vi "ABR Main Panel.vi"(11 "State (in)":T16) -> (3 "State":T16)   [LabVIEW 2020]
uses:
  epl-vi-lib/Utility VIs/Buttons/KCheckmarkBoolean 2.ctl
  CFTS Main Panel SubVIs/CFTS-Experiment State.ctl
  TypeDefs/ABR-Analysis State.ctl
  Threshold Estimation VIs/ABR3-Threshold Estimation Result.ctl
  <vilib>/printing/EasyPrintingControls.llb/layout_options.ctl
  <vilib>/printing/EasyPrintingControls.llb/orientation.ctl
  <vilib>/printing/EasyPrintingControls.llb/panel_scaling_for_page.ctl
  <vilib>/printing/EasyPrintingControls.llb/margins.ctl
  <vilib>/printing/EasyPrintingControls.llb/margin_values.ctl
  <vilib>/printing/EasyPrintingControls.llb/measurement_system.ctl
  <vilib>/printing/EasyPrintingControls.llb/printer_options.ctl
  <vilib>/printing/EasyPrintingControls.llb/printing_method.ctl
  <vilib>/printing/EasyPrintingControls.llb/color_or_monochrome.ctl
  <vilib>/printing/EasyPrintingControls.llb/page_header_options.ctl
  <vilib>/printing/EasyPrintingControls.llb/page_headers.ctl
  <vilib>/printing/EasyPrintingControls.llb/page_header_content_options.ctl
  TypeDefs/ABR-Parameters.ctl
  TypeDefs/ABR-Stimulus.ctl
  TypeDefs/ABR-Response.ctl
  TypeDefs/ABR-Hidden Params.ctl
  Threshold Estimation VIs/ABR3-Threshold Estimation Parameters.ctl
  <vilib>/printing/EasyPrintingControls.llb/contents.ctl
  <vilib>/printing/EasyPrinting.llb/Easy Print VI Panel or Documentation (refnum).vi
  <vilib>/Utility/NIReport.llb/NI_ReportGenerationCore.lvlib
panel:
  out "Thr":string caption="Threshold (dB SPL)"
  in  "layout options":T1={"orientation (unchanged)"=0, "panel scaling for page (unchanged)"=0, "margins"={"override VI margins (false)"=FALSE, "margins (1.00)"={"top"=1.0, "left"=1.0, "right"=1.0, "bottom"=1.0}, "measurement system (default)"=0}, "printer options"={"destination printer name (current)"="", "printing method (unchanged)"=0, "color or monochrome (unchanged)"=0}, "page header options"={"page headers (unchanged)"=0, "page header content options"={"Include VI Name"=TRUE, "Include VI Path"=TRUE, "Include Last Modification Date"=TRUE, "Include Date Printed"=TRUE, "Include Page Number"=TRUE, "Include VI Icon"=TRUE}}} {"page header options"."page headers (unchanged)" items=["Unchanged", "Include page headers", "Do not include page headers"]; "printer options"."color or monochrome (unchanged)" items=["Unchanged", "Color/grayscale", "Monochrome"]; "printer options"."printing method (unchanged)" items=["Unchanged", "Standard", "PostScript", "Bitmap"]; "panel scaling for page (unchanged)" items=["Unchanged", "No Scaling", "Scale front panel to fit"]; "orientation (unchanged)" items=["Unchanged", "portrait", "landscape"]; "margins"."measurement system (default)" items=["Default", "US", "Metric"]; "margins"."margins (1.00)"."right" format="%.2f"; "margins"."margins (1.00)"."bottom" format="%.2f"; "margins"."margins (1.00)"."top" format="%.2f"; "margins"."margins (1.00)"."left" format="%.2f"}
  out "CM":cluster{dbl[], dbl[]}[](graph) caption="\"CM\""
  out "Neural":cluster{dbl[], dbl[]}[](graph)
  in  "NOTES":string
  out "Analysis":T13
  out "finished":errorcluster
  in  "Response":T15={"Gain"=10000, "Averages"=512, "Window (ms)"=8.5, "Thr Fast Steps"=1.5} {"Thr Fast Steps" format="%.2f"; "Window (ms)" format="%.2f"}
  in  "CAP or ABR":enum16{"CAP", "ABR"}(ring)=enum."ABR" caption="Measure what"
  out "MAX SPL":dbl=113.05999755859375 format="%.2f"
  out "SPL":dbl=35.0
  out "User":string
  out "Run #":u16=14
  out "ID #":u16=1
  out "Running":bool
  out "Abort":bool
  in  "Stimulus":T17={"Ear"=enum."Left", "Start (dB)"=20, "Waveform"=enum."TONE PIP", "Stop (dB)"=80, "Frequency (kHz)"=16.0, "Step (dB)"=5, "Rep rate (/sec)"=30.0, "Alternate Polarity"=FALSE} {"Rep rate (/sec)" format="%#_8g"; "Frequency (kHz)" format="%.2f"; "Start (dB)" step=5}
  out "Datafile":path
  in  "Normalize traces":T18=TRUE caption="Normalize individual traces"
  out "CLICK I-O":cluster{dbl[], dbl[]}[](graph)
  in  "START":bool
  in  "RETURN":bool
  in  "STOP":bool
  out "TONE I-O":cluster{dbl[], dbl[]}[](graph)
  # "Response"
  # "Running Average"
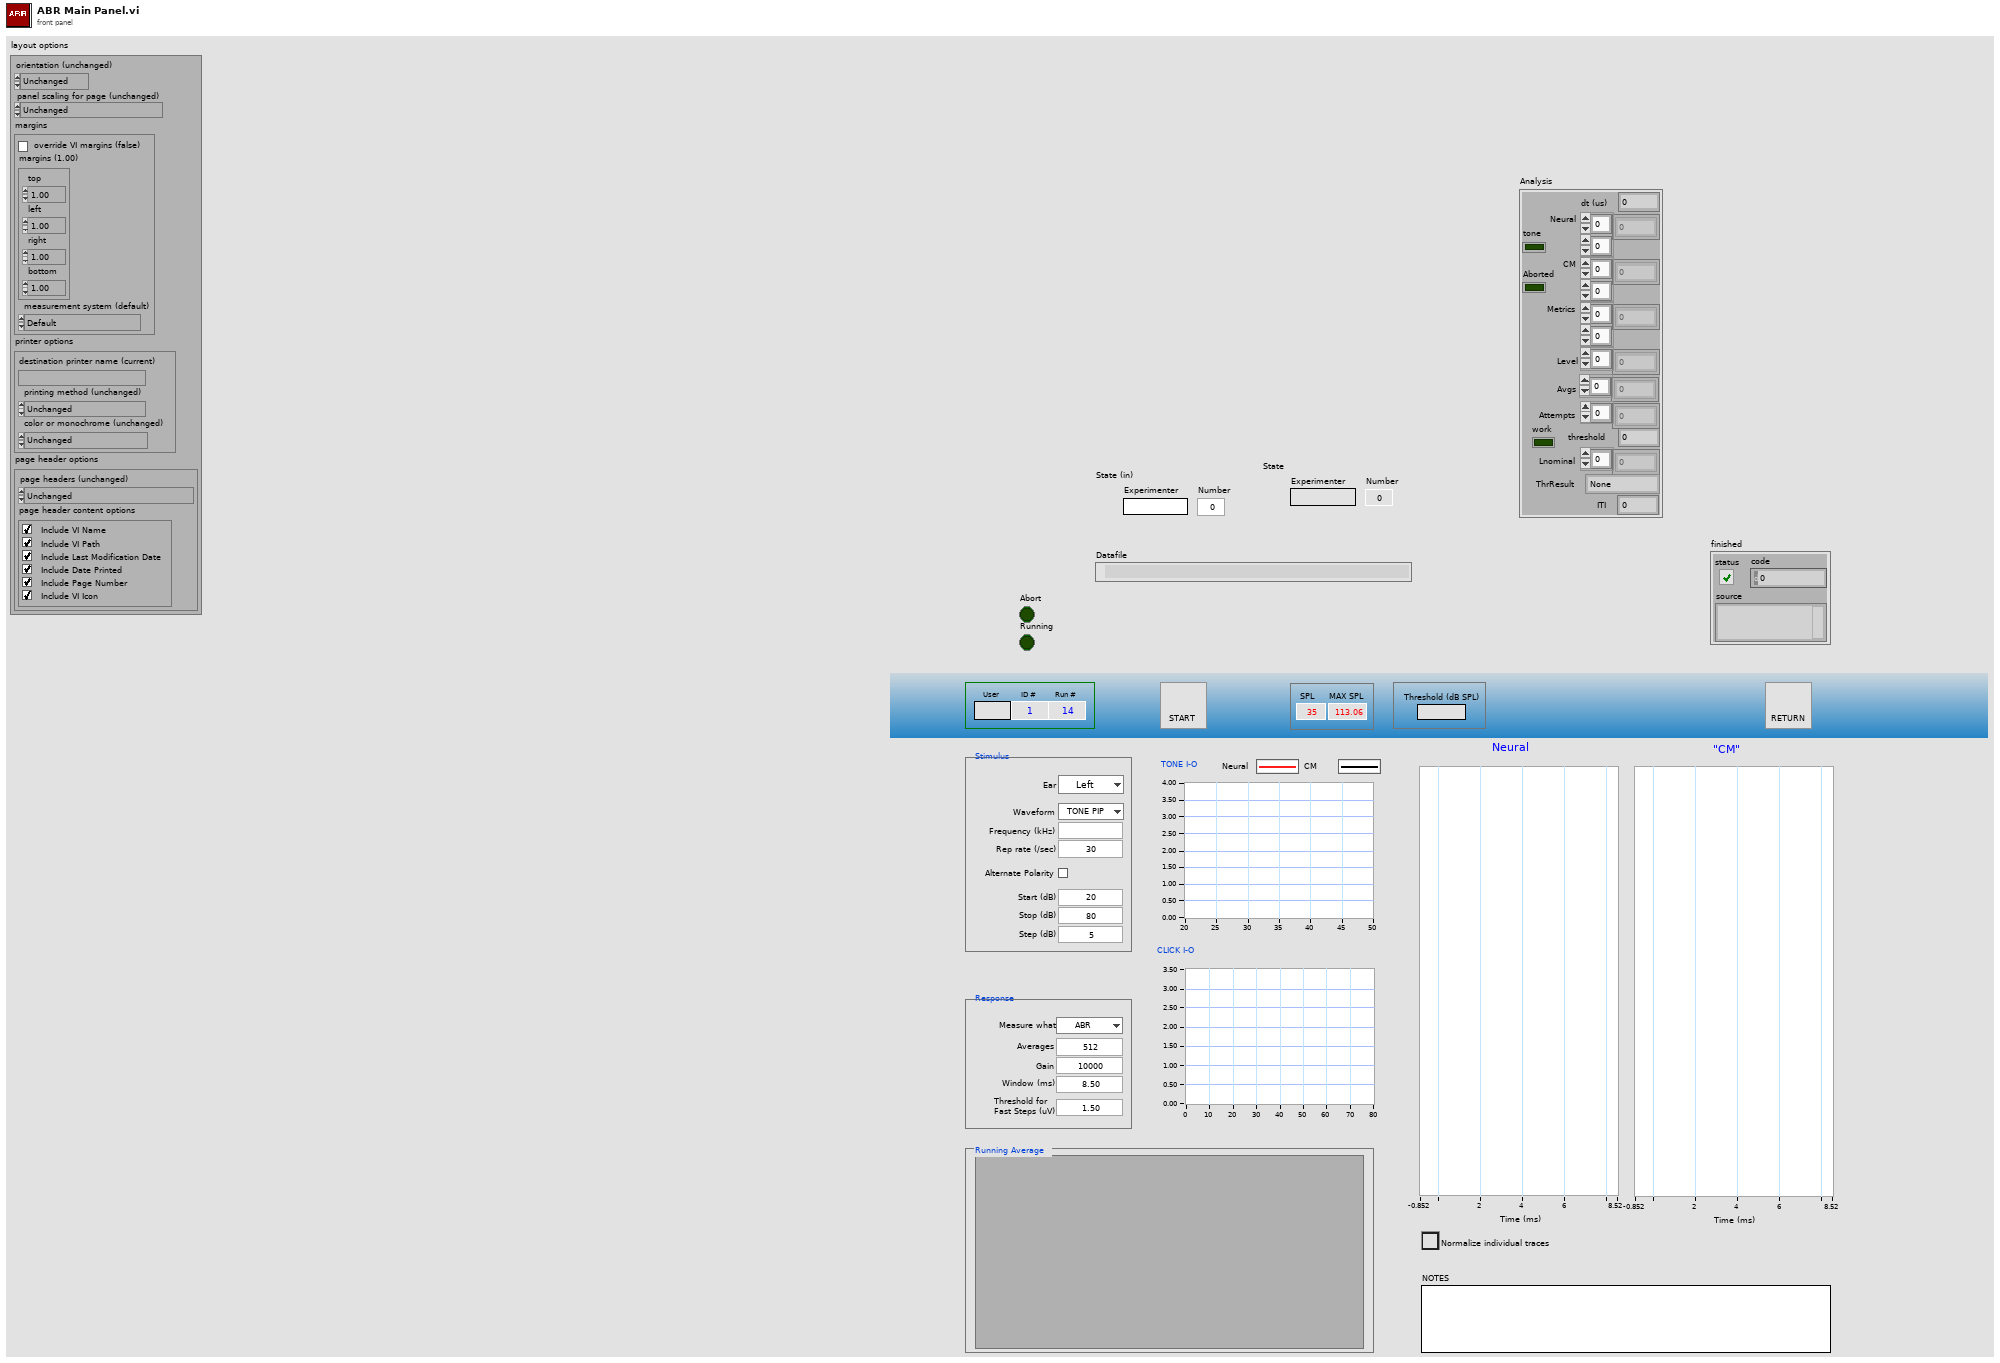
[diagram p1: front panel]
types:
  T1 = typedef "NI_ReportGenerationCore.lvlib/layout_options.ctl" = cluster{"orientation (unchanged)":T2, "panel scaling for page (unchanged)":T3, "margins":T4, "printer options":T7, "page header options":T10}
  T2 = typedef "NI_ReportGenerationCore.lvlib/orientation.ctl" = u16
  T3 = typedef "NI_ReportGenerationCore.lvlib/panel_scaling_for_page.ctl" = u16
  T4 = typedef "NI_ReportGenerationCore.lvlib/margins.ctl" = cluster{"override VI margins (false)":bool, "margins (1.00)":T5, "measurement system (default)":T6}
  T5 = typedef "NI_ReportGenerationCore.lvlib/margin_values.ctl" = cluster{"top":dbl, "left":dbl, "right":dbl, "bottom":dbl}
  T6 = typedef "NI_ReportGenerationCore.lvlib/measurement_system.ctl" = u16
  T7 = typedef "NI_ReportGenerationCore.lvlib/printer_options.ctl" = cluster{"destination printer name (current)":string, "printing method (unchanged)":T8, "color or monochrome (unchanged)":T9}
  T8 = typedef "NI_ReportGenerationCore.lvlib/printing_method.ctl" = u16
  T9 = typedef "NI_ReportGenerationCore.lvlib/color_or_monochrome.ctl" = u16
  T10 = typedef "NI_ReportGenerationCore.lvlib/page_header_options.ctl" = cluster{"page headers (unchanged)":T11, "page header content options":T12}
  T11 = typedef "NI_ReportGenerationCore.lvlib/page_headers.ctl" = u16
  T12 = typedef "NI_ReportGenerationCore.lvlib/page_header_content_options.ctl" = cluster{"Include VI Name":bool, "Include VI Path":bool, "Include Last Modification Date":bool, "Include Date Printed":bool, "Include Page Number":bool, "Include VI Icon":bool}
  T13 = typedef "ABR-Analysis State.ctl" = cluster{"dt (us)":dbl, "Neural":dbl[][], "CM":dbl[][], "Metrics":dbl[][], "Level":dbl[], "Avgs":i32[], "Attempts":i32[], "Aborted":bool, "threshold":dbl, "Lnominal":dbl[], "tone":bool, "work":bool, "ThrResult":T14, "ITI":dbl}
  T14 = typedef "ABR3-Threshold Estimation Result.ctl" = enum16{"None", "Power", "Sigmoid", "Power (noisy)", "Suprathreshold", "Invalid"}
  T15 = cluster{"Gain":i32, "Averages":i32, "Window (ms)":sgl, "Thr Fast Steps":sgl}
  T16 = typedef "CFTS-Experiment State.ctl" = cluster{"Experimenter":string, "Number":u32, "Right":string, "Left":string, "Data Folder":path, "State File":path, "Version Info":string, "End Exposure Time":dbl, "Exposure Duration":string, "Run #":cluster{"CAP":i16, "ABR":i16, "DP":i16, "VsEP":i16, "MeasSeq":i16, "SubSeq":i16, "SFOAE":i16}}
  T17 = cluster{"Ear":enum16{"Right", "Left"}, "Start (dB)":i32, "Waveform":enum16{"TONE PIP", "CLICK"}, "Stop (dB)":i32, "Frequency (kHz)":ext, "Step (dB)":i32, "Rep rate (/sec)":dbl, "Alternate Polarity":bool}
  T18 = typedef "KCheckmarkBoolean 2.ctl" = bool
  T19 = typedef "ABR3-Threshold Estimation Parameters.ctl" = cluster{"Tmin (ms)":dbl, "Tmax (ms)":dbl, "CC criterion":dbl, "adjR2 criterion":dbl}
  T20 = typedef "ABR-Parameters.ctl" = cluster{"CAP or ABR":enum16{"CAP", "ABR"}, "Stimulus":T21, "Response":T22, "Hidden":T23, "Version":i32}
  T21 = typedef "ABR-Stimulus.ctl" = cluster{"Ear":enum16{"Right", "Left", "Bone"}, "Start (dB)":i32, "Waveform":enum16{"TONE PIP", "CLICK"}, "Stop (dB)":i32, "Frequency (kHz)":ext, "Step (dB)":i32, "Rep rate (/sec)":dbl, "Alternate Polarity":bool}
  T22 = typedef "ABR-Response.ctl" = cluster{"Gain":i32, "Averages":i32, "Window (ms)":sgl, "Thr Fast Steps":sgl}
  T23 = typedef "ABR-Hidden Params.ctl" = cluster{"AI Samp Rate Hz":dbl, "AO Samp Rate Hz":dbl, "Duration (ms)":dbl, "Ramp (ms)":dbl, "Click width (us)":dbl, "ITI":enum16{"Rate", "Interval"}, "Save raw":bool}
  T24 = cluster{"Params":T20, "Threshold Estimation":T19}
  T25 = cluster{"TONE I-O":refnum<vi>, "Neural":refnum<vi>, "CM":refnum<vi>, "CLICK I-O":refnum<vi>}
  T26 = typedef "NI_ReportGenerationCore.lvlib/contents.ctl" = u16
  T27 = typedef "ABR3-Threshold Estimation Work.ctl" = cluster{"Threshold":dbl, "Criterion":dbl, "graphs":cluster{"X":dbl[], "Y":dbl[]}[], "Power2":string, "Sigmoid":string, "Result":T14}
  T28 = cluster{"Params":T20, "Threshold Estimation Out":T19}
  T29 = typedef "ABR-Runtime Data.ctl" = cluster{"AO Channels":i32[], "Ceiling":dbl, "Threshold":dbl, "Crossed?":bool, "Step":dbl, "Stop":i32, "Avgs":i32, "Level":dbl, "AI Npts":i32, "Doubled?":bool, "AO Npts":i32, "AltPol":bool, "dt":dbl, "gain":dbl, "reps/buffer":i32, "NWinPts":i32, "Save raw":bool}
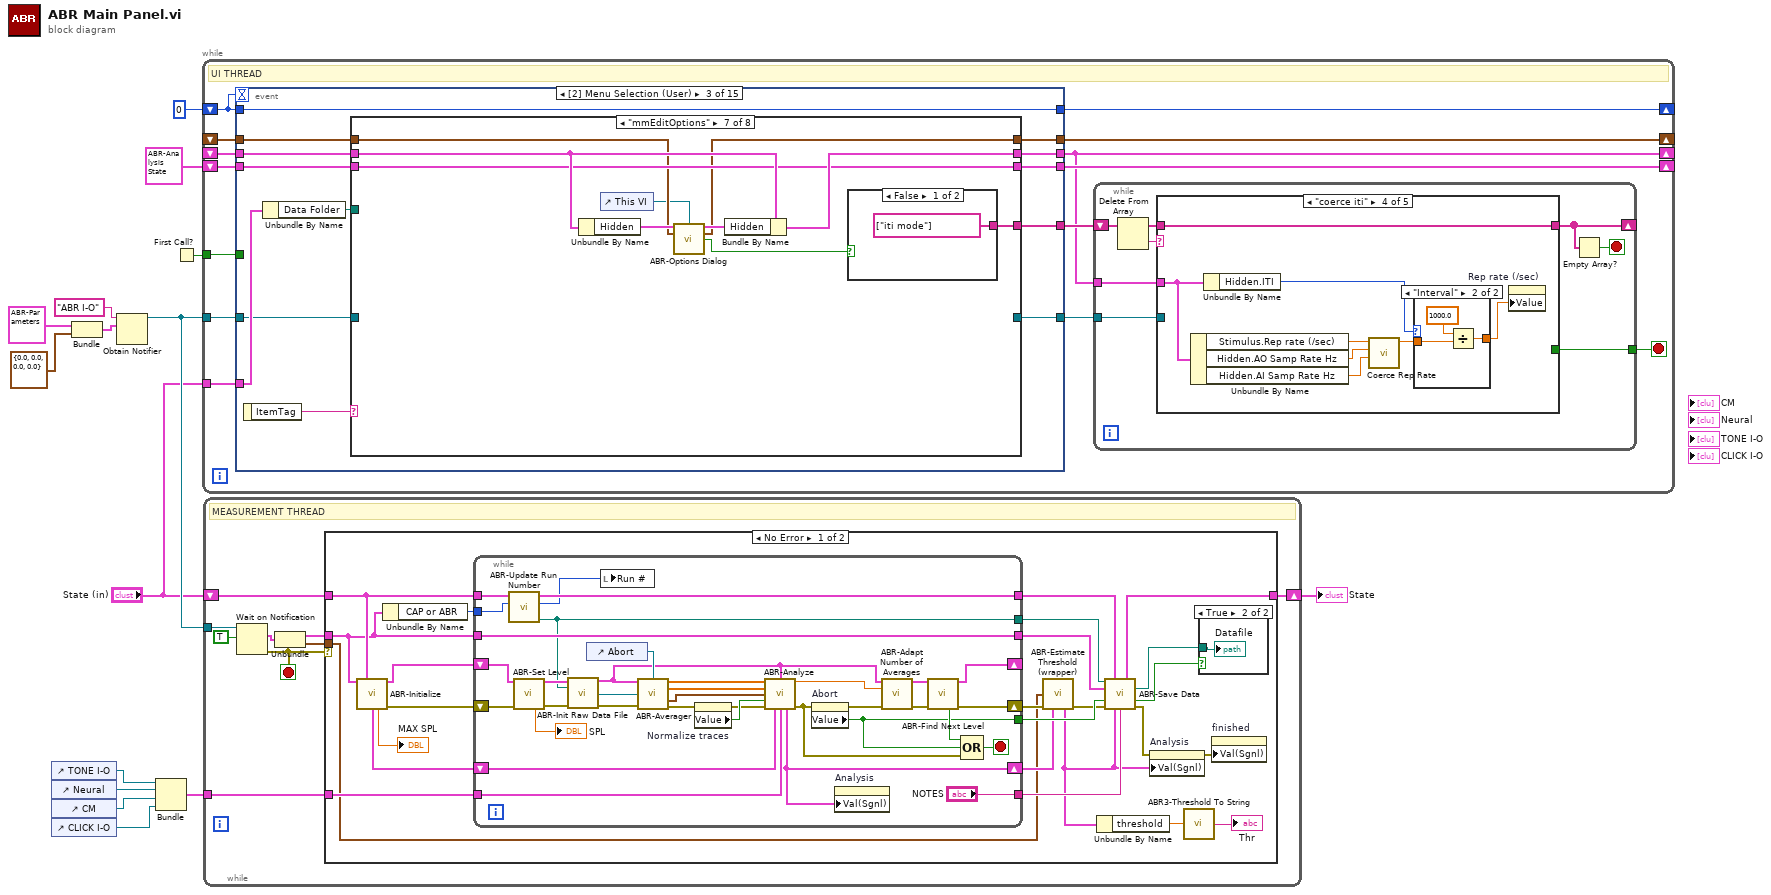
[diagram p0: block diagram]
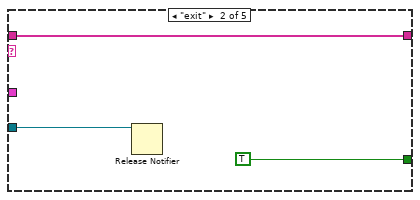
[diagram p5: hidden frame]
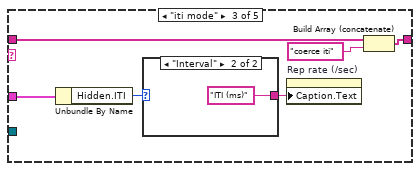
[diagram p6: hidden frame]
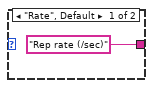
[diagram p7: hidden frame]
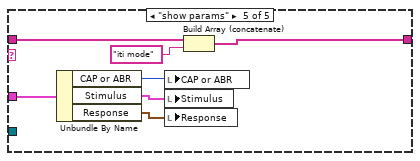
[diagram p9: hidden frame]
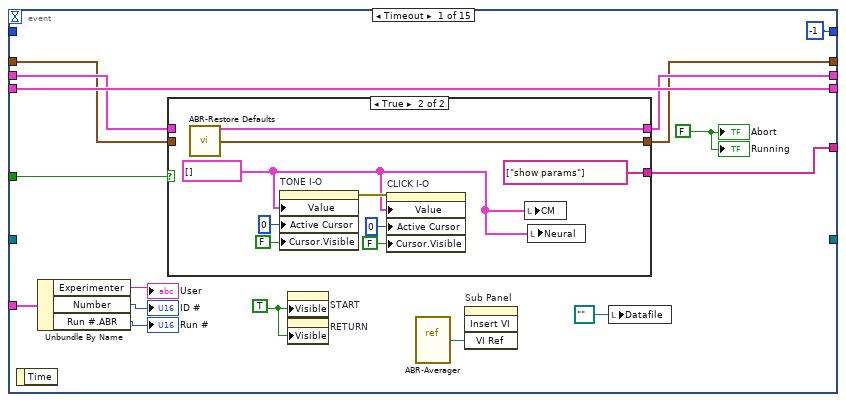
[diagram p10: hidden frame]
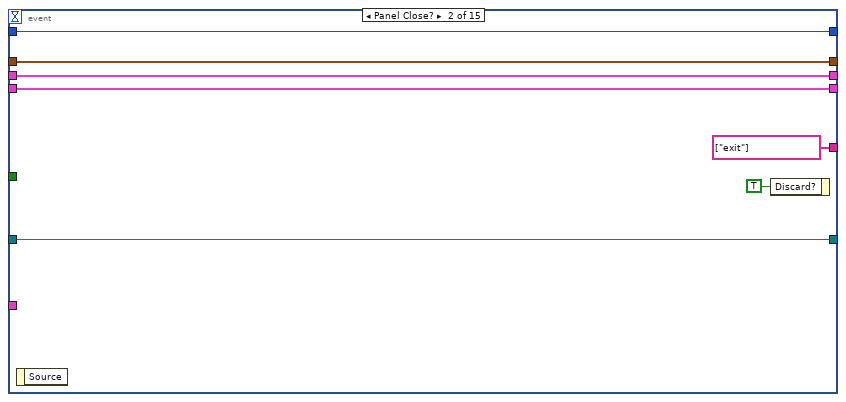
[diagram p12: hidden frame]
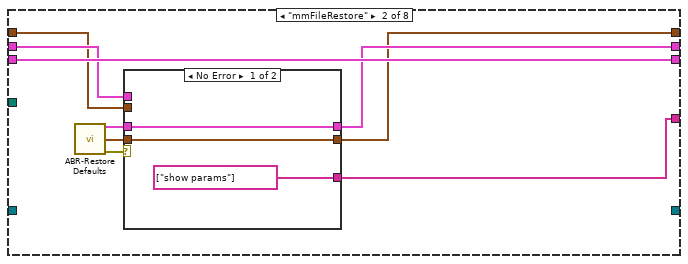
[diagram p14: hidden frame]
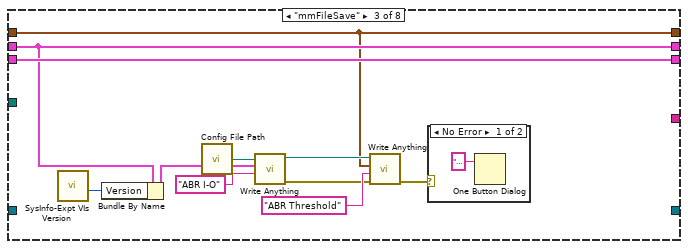
[diagram p16: hidden frame]
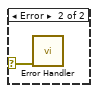
[diagram p17: hidden frame]
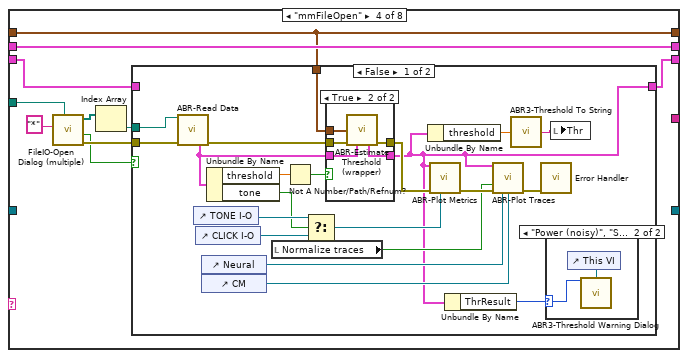
[diagram p18: hidden frame]
diagram:
  n1 = control-ref of="TONE I-O"() -> (w6:refnum<vi>)
  n2 = control-ref of="Neural"() -> (w8:refnum<vi>)
  n3 = control-ref of="CM"() -> (w7:refnum<vi>)
  n4 = control-ref of="CLICK I-O"() -> (w5:refnum<vi>)
  n5 = Bundle("Params"=T20 {"CAP or ABR"=enum."ABR", "Stimulus"={"Ear"=enum."Left", "Start (dB)"=0, "Waveform"=enum."TONE PIP", "Stop (dB)"=30, "Frequency (kHz)"=16.0, "Step (dB)"=5, "Rep rate (/sec)"=30.0, "Alternate Polarity"=FALSE}, "Response"={"Gain"=10000, "Averages"=512, "Window (ms)"=8.5, "Thr Fast Steps"=8.5}, "Hidden"={"AI Samp Rate Hz"=25000.0, "AO Samp Rate Hz"=100000.0, "Duration (ms)"=5.0, "Ramp (ms)"=0.5, "Click width (us)"=0.0, "ITI"=enum."Rate", "Save raw"=FALSE}, "Version"=0}, "Threshold Estimation"=T19 {"Tmin (ms)"=0.0, "Tmax (ms)"=0.0, "CC criterion"=0.0, "adjR2 criterion"=0.0}) -> (w1:T24)  [unwired: 1 in]
  n6 = Obtain Notifier(name (unnamed)="ABR I-O", notification data type=w1) -> (notifier out=w15:refnum<notifier>)  [unwired: 2 in, 2 out]
  n7 = Bundle("TONE I-O"=w6, "Neural"=w8, "CM"=w7, "CLICK I-O"=w5) -> (w9:T25)  [unwired: 1 in]
  n8 = First Call?() -> (First Call?: T/F=w13:bool)
  n9 = while {
    tunnel: w15 -> [w29]
    shift-right: [w26] -> _
    shift-left: 0 -> [w27]
    tunnel: w13 -> [w28]
    shift-right: [w17] -> _
    shift-left: _ -> [w25]
    tunnel: "State (in)" -> [w24]
    shift-right: [w22] -> _
    shift-left: T13 {"dt (us)"=0.0, "Neural"=[], "CM"=[], "Metrics"=[], "Level"=[], "Avgs"=[], "Attempts"=[], "Aborted"=FALSE, "threshold"=0.0, "Lnominal"=[], "tone"=FALSE, "work"=FALSE, "ThrResult"=enum."None", "ITI"=0.0} ("Analysis") -> [w23]
    shift-right: [w16] -> _
    shift-left: _ -> [w21]
    stop <- w18 stop-if-true
    # "UI THREAD"
    n10 = event shown="[2] Menu Selection (User)" {
      selector: _ -> [_ _ _ _ _ _ _ _ _ _ _ _ _ _ _]
      dyn-events: _ -> [_ _ _ _ _ _ _ _ _ _ _ _ _ _ _]
      timeout: w27 -> [_ _ _ _ _ _ _ _ _ _ _ _ _ _ _]
      tunnel: w29 -> [_ w96 w103 _ _ w230 w239 _ _ _ _ _ _ _ _]
      tunnel: [_ w96 w104 _ _ w230 _ _ _ _ _ _ _ _ _] -> w19
      tunnel: [-1 w102 w115 w218 w224 w229 w236 w243 w261 w267 w277 w299 w311 w317 w321] -> w26
      tunnel: w28 -> [w74 _ _ _ _ _ _ _ _ _ _ _ _ _ _]
      tunnel: w27 -> [_ w102 w115 w218 w224 w229 w236 w243 w261 w267 w277 w299 w311 w317 w321]
      tunnel: w25 -> [w73 w101 w111 w217 w223 w228 w232 w242 w258 w266 w276 w295 w310 w316 w320]
      tunnel: [w72 w101 w110 w217 w223 w228 w232 w242 w258 w266 w276 w298 w309 w315 w320] -> w17
      tunnel: w24 -> [w76 _ w113 _ _ _ _ _ _ _ _ _ _ _ _]
      tunnel: w23 -> [w75 w100 w109 w216 w222 w227 w235 w241 w247 w265 w275 w297 w307 w313 _]
      tunnel: [w75 w100 w108 w216 w221 w227 w235 w241 w247 w265 w275 w297 w307 w313 w319] -> w22
      tunnel: [w71 w98 w106 w213 w219 w226 w231 w240 w248 w264 w274 w296 w306 w312 w318] -> w16
      tunnel: w21 -> [w70 w98 w107 w213 w219 w226 w231 w240 w248 w264 w274 w296 w306 w312 w318]
      tunnel: [w69 string[] ["exit"] w105 _ _ string[] ["exit"] _ _ _ _ _ string[] ["coerce iti"] _ _ _] -> w20
      event Timeout {
        w79 = FALSE ("quitting")
        w80 = TRUE
        n11 = event-data() -> ()  [unwired: 1 in, 1 out]
        n12 = Unbundle By Name(w76) -> ("Experimenter"=→"User":string, "Number"=→"ID #":u32, "Run #.ABR"=→"Run #":i16)
        n13 = case shown="True" w74 {
          tunnel: w73 -> [w86 _]
          tunnel: [w86 w95] -> w72
          tunnel: [w85 w88] -> w71
          tunnel: w70 -> [w85 _]
          tunnel: [_ string[] ["show params"]] -> w69
          frame False {
          }
          frame True {
            w89 = cluster{dbl[], dbl[]}[] [] ("TONE I-O")
            n14 = call "ABR-Restore Defaults.vi"() -> ("Params"=w95:T20, "Threshold Estimation"=w88:T19)  [unwired: 13 in, 1 out]
            n15 = property on="TONE I-O" class="XYGraph (strict)"("Value"=w89, "Active Cursor"=u32 0, "Cursor.Visible"=FALSE) -> (error out=w92:errorcluster)  [unwired: 2 in, 1 out]
            n16 = property on="CLICK I-O" class="XYGraph (strict)"(error in=w92, "Value"=w89, "Active Cursor"=u32 0, "Cursor.Visible"=FALSE) -> ()  [unwired: 1 in, 2 out]
            n17 = local write "CM"(w89) -> ()
            n18 = local write "Neural"(w89) -> ()
          }
        }
        n19 = property on="START" class="Bool"("Visible"=w80) -> ()  [unwired: 2 in, 2 out]
        n20 = property on="RETURN" class="Bool"("Visible"=w80) -> ()  [unwired: 2 in, 2 out]
        n21 = vi-ref "ABR-Averager.vi"() -> (w83:refnum<vi>)
        n22 = invoke on="Sub Panel" class="SubPanel" method="Insert VI"("VI Ref"=w83) -> ()  [unwired: 3 in, 4 out]
        n23 = local write "Datafile"(path "" ("Datafile path")) -> ()
        "Abort" <- w79
        "Running" <- w79
      }
      event Panel Close? {
        n24 = event-data() -> ()  [unwired: 1 in, 1 out]
        n25 = event-data("Discard?"=TRUE) -> ()  [unwired: 1 in, 1 out]
      }
      event Menu Selection (User) {
        n26 = event-data() -> ("ItemTag"=w114:string)  [unwired: 1 in]
        n27 = Unbundle By Name(w113) -> ("Data Folder"=w112:path)
        n28 = case shown="\"mmEditOptions\"" w114 {
          tunnel: w111 -> [w118 w124 w141 w149 w192 w197 w204 w212]
          tunnel: [w118 w123 w141 w149 w192 w197 w205 w212] -> w110
          tunnel: w112 -> [_ _ _ w150 _ _ _ _]
          tunnel: w109 -> [w117 w127 w143 w148 w188 w196 w203 w210]
          tunnel: [w117 w127 w143 w147 w188 w196 w203 w210] -> w108
          tunnel: w107 -> [w116 w121 w135 w146 w187 w195 w202 w209]
          tunnel: [w116 w120 w135 w146 w187 w195 w201 w209] -> w106
          tunnel: [_ w119 _ _ _ string[] ["exit"] w198 _] -> w105
          tunnel: [_ _ _ _ _ w193 _ _] -> w104
          tunnel: w103 -> [_ _ _ _ _ w193 _ _]
          frame "False", Default {
          }
          frame "mmFileRestore" {
            n29 = call "ABR-Restore Defaults.vi"() -> ("Params"=w125:T20, "Threshold Estimation"=w122:T19, "error out"=w126:errorcluster)  [unwired: 13 in]
            n30 = case shown="No Error" w126 {
              tunnel: w125 -> [w130 _]
              tunnel: w124 -> [_ w132]
              tunnel: [w130 w132] -> w123
              tunnel: w122 -> [w129 _]
              tunnel: w121 -> [_ w131]
              tunnel: [w129 w131] -> w120
              tunnel: [string[] ["show params"] _] -> w119
              frame No Error {
              }
              frame Error {
              }
            }
          }
          frame "mmFileSave" {
            n31 = call "SysInfo-Expt VIs Version.vi"() -> ("Expt VIs Version out"=w133:i32)  [unwired: 11 in]
            n32 = Bundle By Name(cluster=w141, "Version"=w133) -> (w134:T20)
            n33 = call "Config File Path.vi"() -> ("Default config file name"=w142:path)  [unwired: 1 in]
            n34 = call "Write Anything.vi"("Section Name (Name of \"Anything\")"="ABR I-O" ("Section Name (Name of \"Anything\")"), "Anything"=w134, "Path (dialog)"=w142) -> ("Error Out"=w137:errorcluster, "Path out"=w138:path)  [unwired: 7 in]
            n35 = call "Write Anything.vi"("Error In"=w137, "Section Name (Name of \"Anything\")"="ABR Threshold" ("Section Name (Name of \"Anything\")"), "Anything"=w135, "Path (dialog)"=w138) -> ("Error Out"=w136:errorcluster)  [unwired: 6 in, 1 out]
            n36 = case shown="No Error" w136 {
              selector: w136 -> [_ w145]
              frame No Error {
                n37 = One Button Dialog(message="Defaults saved.") -> ()  [unwired: 1 in, 1 out]
              }
              frame Error {
                n38 = call "Error Handler.vi"("error in (no error)"=w145) -> ()  [unwired: 13 in, 2 out]
              }
            }
          }
          frame "mmFileOpen" {
            n39 = call "FileIO-Open Dialog (multiple).vi"("Default Folder"=w150, "pattern (all files)"="*") -> ("error out"=w155:errorcluster, "cancelled"=w151:bool, "Paths"=w154:path[])  [unwired: 7 in]
            n40 = Index Array(array=w154) -> (element=w153:path)  [unwired: 1 in]
            n41 = case shown="False" w151 {
              tunnel: w155 -> [w176 _]
              tunnel: w153 -> [w175 _]
              tunnel: w148 -> [_ w186]
              tunnel: [w157 w186] -> w147
              tunnel: w146 -> [w158 _]
              frame False {
                n42 = call "ABR-Read Data.vi"("Path"=w175, "error in (no error)"=w176) -> ("Analysis"=w161:T13, "error out"=w163:errorcluster)  [unwired: 8 in, 4 out]
                n43 = control-ref of="TONE I-O"() -> (w168:refnum<vi>)
                n44 = control-ref of="CLICK I-O"() -> (w169:refnum<vi>)
                n45 = control-ref of="Neural"() -> (w172:refnum<vi>)
                n46 = control-ref of="CM"() -> (w171:refnum<vi>)
                n47 = Unbundle By Name(w161) -> ("threshold"=w165:dbl, "tone"=w166:bool)
                n48 = local read "Normalize traces"() -> (w173:T18)
                n49 = Not A Number/Path/Refnum?(number/path/refnum=w165) -> (NaN/Path/Refnum?=w164:bool)
                n50 = Select(t=w168, s=w166, f=w169) -> (s? t:f=w167:refnum<vi>)
                n51 = case shown="True" w164 {
                  tunnel: w163 -> [w180 w185]
                  tunnel: [w180 w184] -> w162
                  tunnel: w161 -> [w179 w183]
                  tunnel: [w179 w182] -> w157
                  tunnel: w158 -> [_ w181]
                  frame False {
                  }
                  frame True {
                    n52 = call "ABR-Estimate Threshold (wrapper).vi"("Threshold Estimation"=w181, "error in (no error)"=w185, "Analysis (in)"=w183) -> ("Analysis (out)"=w182:T13, "error out"=w184:errorcluster)  [unwired: 10 in, 1 out]
                  }
                }
                n53 = Unbundle By Name(w157) -> ("threshold"=w160:dbl)
                n54 = call "ABR-Plot Metrics.vi"("Analysis"=w157, "error in (no error)"=w162, "I-O"=w167) -> ("error out"=w174:errorcluster)  [unwired: 12 in]
                n55 = Unbundle By Name(w157) -> ("ThrResult"=w156:T14)
                n56 = call "ABR-Plot Traces.vi"("Analysis"=w157, "Normalize individual?"=w173, "error in (no error)"=w174, "Neural Ref"=w172, "CM Ref"=w171) -> ("error out"=w170:errorcluster)  [unwired: 10 in]
                n57 = call "ABR3-Threshold To String.vi"("Threshold"=w160) -> ("String"=w159:string)
                n58 = call "Error Handler.vi"("error in (no error)"=w170) -> ()  [unwired: 13 in, 2 out]
                n59 = case shown="\"Power (noisy)\", \"Suprathreshold\"" w156 {
                  selector: w156 -> [_ w178]
                  frame "None", Default {
                  }
                  frame "Power (noisy)", "Suprathreshold" {
                    n60 = control-ref of="This VI"() -> (w177:refnum<vi>)
                    n61 = call "ABR3-Threshold Warning Dialog.vi"("Result"=w178, "Parent VI"=w177) -> ()  [unwired: 14 in]
                  }
                }
                n62 = local write "Thr"(w159) -> ()
              }
              frame True {
              }
            }
          }
          frame "mmFilePrint" {
            w191 = T26 1 items=["Complete front panel", "Visible portion of front panel", "Icon, description, panel and diagram", "Documentation: Using the panel", "Documentation: Using as a subVI", "Documentation: Complete", "Documentation: Custom"] ("contents (complete front panel)")
            n63 = control-ref of="This VI"() -> (w189:refnum<vi>)
            n64 = call-poly <vilib>:"Easy Print VI Panel or Documentation.vi"("layout options"="layout options", "contents (complete front panel)"=w191, "VI reference"=w189) -> ()  [unwired: 7 in, 2 out]
          }
          frame "mmFileExit" {
          }
          frame "mmEditOptions" {
            n65 = Unbundle By Name(w204) -> ("Hidden"=w207:T23)
            n66 = control-ref of="This VI"() -> (w200:refnum<vi>)
            n67 = call "ABR-Options Dialog.vi"("Hidden"=w207, "Parent VI"=w200, "Threshold Estimation In"=w202) -> ("Cluster out"=w206:T23, "Threshold Estimation Out"=w201:T19, "Canceled?"=w199:bool)  [unwired: 10 in]
            n68 = Bundle By Name(cluster=w204, "Hidden"=w206) -> (w205:T20)
            n69 = case shown="False" w199 {
              tunnel: [string[] ["iti mode"] _] -> w198
              frame False {
              }
              frame True {
              }
            }
          }
          frame "mmHelpManual" {
            n70 = call "CFTS-Open Help Topic.vi"("Topic Keyword"="ABR/CAP") -> ()  [unwired: 14 in, 1 out]
          }
        }
      }
      event "CLICK I-O", "TONE I-O": Shortcut Menu Activation? {
        n71 = event-data() -> ()  [unwired: 1 in, 1 out]
        n72 = Unbundle By Name(w216) -> ("Neural"=w215:dbl[][])
        n73 = Empty Array?(array=w215) -> (empty?=w214:bool)
        n74 = event-data("Discard?"=w214) -> ()  [unwired: 1 in, 1 out]
      }
      event "CLICK I-O", "TONE I-O": Shortcut Menu Selection (User) {
        n75 = event-data() -> ()  [unwired: 1 in, 1 out]
        n76 = call "ABR-Estimate Threshold (wrapper).vi"("Analysis (in)"=w222) -> ("Work"=w220:T27, "Analysis (out)"=w221:T13)  [unwired: 12 in, 1 out]
        n77 = call "ABR3-Show Threshold Estimation Work.vi"("work"=w220) -> ()  [unwired: 15 in]
      }
      event "RETURN": Value Change {
        n78 = event-data() -> ()  [unwired: 1 in, 1 out]
      }
      event "START": Value Change {
        w237 = FALSE ("ABI Abort")
        n79 = event-data() -> ()  [unwired: 1 in, 1 out]
        n80 = Bundle("Params"=w232, "Threshold Estimation Out"=w231) -> (w233:T28)  [unwired: 1 in]
        n81 = Send Notification(notification=w233, notifier=w239) -> ()  [unwired: 1 in, 2 out]
        n82 = local write "NOTES"("" ("NOTES")) -> ()
        n83 = local write "Abort"(w237) -> ()
        n84 = property on="RETURN" class="Bool"("Visible"=w237) -> ()  [unwired: 2 in, 2 out]
        n85 = property on="START" class="Bool"("Visible"=w237) -> ()  [unwired: 2 in, 2 out]
        n86 = local write "Running"(TRUE ("Running")) -> ()
      }
      event "STOP": Value Change {
        n87 = event-data() -> ()  [unwired: 1 in, 1 out]
        n88 = local write "Abort"(TRUE ("Stopping")) -> ()
      }
      event "finished": Value Change {
        w259 = TRUE
        n89 = event-data() -> ("NewVal"=w257:errorcluster)  [unwired: 1 in]
        n90 = Unbundle By Name(w247) -> ("tone"=w256:bool)
        n91 = call "Error Handler.vi"("error in (no error)"=w257) -> ()  [unwired: 13 in, 2 out]
        n92 = control-ref of="TONE I-O"() -> (w254:refnum<vi>)
        n93 = control-ref of="CLICK I-O"() -> (w253:refnum<vi>)
        n94 = control-ref of="Neural"() -> (w251:refnum<vi>)
        n95 = control-ref of="CM"() -> (w252:refnum<vi>)
        n96 = local read "Normalize traces"() -> (w250:T18)
        n97 = Select(t=w254, s=w256, f=w253) -> (s? t:f=w255:refnum<vi>)
        n98 = call "ABR-Plot Metrics.vi"("Analysis"=w247, "I-O"=w255) -> ("error out"=w249:errorcluster)  [unwired: 13 in]
        n99 = Unbundle By Name(w247) -> ("ThrResult"=w246:T14)
        n100 = call "ABR-Plot Traces.vi"("Analysis"=w247, "Normalize individual?"=w250, "error in (no error)"=w249, "Neural Ref"=w251, "CM Ref"=w252) -> ("error out"=w245:errorcluster)  [unwired: 10 in]
        n101 = case shown="\"Power (noisy)\", \"Suprathreshold\"" w246 {
          selector: w246 -> [_ w263]
          tunnel: w245 -> [_ _]
          frame "None", Default {
          }
          frame "Power (noisy)", "Suprathreshold" {
            n102 = control-ref of="This VI"() -> (w262:refnum<vi>)
            n103 = call "ABR3-Threshold Warning Dialog.vi"("Result"=w263, "Parent VI"=w262) -> ()  [unwired: 14 in]
          }
        }
        n104 = call "Beeper.vi"() -> ()  [unwired: 5 in, 1 out]
        n105 = property on="RETURN" class="Bool"("Visible"=w259) -> ()  [unwired: 2 in, 2 out]
        n106 = property on="START" class="Bool"("Visible"=w259) -> ()  [unwired: 2 in, 2 out]
        n107 = local write "Running"(FALSE ("Running")) -> ()
      }
      event Value Change {
        n108 = event-data() -> ("NewVal"=w269:T18)  [unwired: 1 in]
        n109 = case shown="False" FALSE {
          tunnel: w269 -> [w273 _]
          tunnel: w265 -> [w272 _]
          frame False {
            n110 = control-ref of="Neural"() -> (w271:refnum<vi>)
            n111 = control-ref of="CM"() -> (w270:refnum<vi>)
            n112 = call "ABR-Plot Traces.vi"("Analysis"=w272, "Normalize individual?"=w273, "Neural Ref"=w271, "CM Ref"=w270) -> ()  [unwired: 11 in, 1 out]
          }
          frame True {
          }
        }
      }
      event "NOTES": Value Change {
        n113 = event-data() -> ("NewVal"=w279:string)  [unwired: 1 in]
        n114 = local read "Running"() -> (w285:bool)
        n115 = local read "Datafile"() -> (w280:path)
        n116 = Not(x=w285) -> (.not. x?=w283:bool)
        n117 = Empty String/Path?(string/path=w280) -> (empty?=w284:bool)
        n118 = Not(x=w284) -> (.not. x?=w282:bool)
        n119 = And(x=w282, y=w283) -> (x .and. y?=w281:bool)
        n120 = case shown="True" w281 {
          tunnel: w280 -> [_ w289]
          tunnel: w279 -> [_ w288]
          tunnel: "Add notes to data file?" ("message") -> [_ w287]
          frame False {
          }
          frame True {
            n121 = Two Button Dialog(message=w287) -> (T button?=w286:bool)  [unwired: 2 in]
            n122 = case shown="True" w286 {
              tunnel: w289 -> [_ w290]
              tunnel: w288 -> [_ _]
              frame False {
              }
              frame True {
                n123 = call "ABR-Insert Notes.vi"("path"=w290) -> ()  [unwired: 13 in, 2 out]
              }
            }
          }
        }
      }
      event "Stimulus": Value Change {
        n124 = event-data() -> ()  [unwired: 1 in, 1 out]
        n125 = Unbundle By Name(w295) -> ("Hidden.ITI"=w294:enum16{"Rate", "Interval"})
        n126 = case shown="\"Interval\"" w294 {
          tunnel: [w300 w301] -> w293
          tunnel: "Stimulus" -> [w300 w303]
          frame "Rate", Default {
          }
          frame "Interval" {
            n127 = Unbundle By Name(w303) -> ("Rep rate (/sec)"=w305:dbl)
            n128 = Divide(x=1000.0, y=w305) -> (x/y=w302:dbl)
            n129 = Bundle By Name(cluster=w303, "Rep rate (/sec)"=w302) -> (w301:T17)
          }
        }
        n130 = Bundle By Name(cluster=w295, "Stimulus"=w293) -> (w298:T20)
      }
      event "CAP or ABR": Value Change {
        n131 = event-data() -> ()  [unwired: 1 in, 1 out]
        n132 = Bundle By Name(cluster=w310, "CAP or ABR"="CAP or ABR") -> (w309:T20)
      }
      event "Response": Value Change {
        n133 = event-data() -> ()  [unwired: 1 in, 1 out]
        n134 = Bundle By Name(cluster=w316, "Response"="Response") -> (w315:T20)
      }
      event Value Change {
        n135 = event-data() -> ("NewVal"=w319:T13)  [unwired: 1 in]
      }
    }
    n136 = while {
      shift-right: [w34] -> _
      shift-left: w20 -> [w37]
      tunnel: w19 -> [w32]
      tunnel: [w31] -> w18
      tunnel: w17 -> [w30]
      stop <- w33 stop-if-true
      n137 = Delete From Array(array=w37) -> (deleted portion=w35:string, array with subset deleted=w36:string[])  [unwired: 2 in]
      n138 = case shown="\"coerce iti\"" w35 {
        tunnel: w36 -> [w38 w41 w47 w57 w68]
        tunnel: [w38 w41 w43 w57 w63] -> w34
        tunnel: w32 -> [_ w40 _ _ _]
        tunnel: [_ TRUE _ _ _] -> w31
        tunnel: w30 -> [_ _ w46 w55 w64]
        frame "", Default {
        }
        frame "exit" {
          n139 = Release Notifier(notifier=w40) -> ()  [unwired: 2 in, 3 out]
        }
        frame "iti mode" {
          n140 = Unbundle By Name(w46) -> ("Hidden.ITI"=w45:enum16{"Rate", "Interval"})
          n141 = case shown="\"Interval\"" w45 {
            tunnel: ["Rep rate (/sec)" ("Caption.Text") "ITI (ms)" ("Caption.Text")] -> w44
            frame "Rate", Default {
            }
            frame "Interval" {
            }
          }
          n142 = property on="Rep rate (/sec)" class="DigNum (strict)"("Caption.Text"=w44) -> ()  [unwired: 2 in, 2 out]
          n143 = Build Array (concatenate)(w47, "coerce iti") -> (w43:string[])
        }
        frame "coerce iti" {
          n144 = Unbundle By Name(w55) -> ("Stimulus.Rep rate (/sec)"=w54:dbl, "Hidden.AO Samp Rate Hz"=w53:dbl, "Hidden.AI Samp Rate Hz"=w52:dbl)
          n145 = Unbundle By Name(w55) -> ("Hidden.ITI"=w56:enum16{"Rate", "Interval"})
          n146 = call "Coerce Rep Rate.vi"("AI sampling rate (Hz)"=w52, "AO sampling rate (Hz)"=w53, "Rep rate (Hz)"=w54) -> ("Coerced rep rate (Hz)"=w51:dbl)  [unwired: 5 in, 3 out]
          n147 = case shown="\"Interval\"" w56 {
            tunnel: w51 -> [w58 w61]
            tunnel: [w58 w60] -> w50
            frame "Rate", Default {
            }
            frame "Interval" {
              n148 = Divide(x=1000.0, y=w61) -> (x/y=w60:dbl)
            }
          }
          n149 = property on="Rep rate (/sec)" class="DigNum (strict)"("Value"=w50) -> ()  [unwired: 2 in, 2 out]
        }
        frame "show params" {
          n150 = Unbundle By Name(w64) -> ("CAP or ABR"=w67:enum16{"CAP", "ABR"}, "Stimulus"=w66:T21, "Response"=w65:T22)
          n151 = local write "CAP or ABR"(w67) -> ()
          n152 = local write "Stimulus"(w66) -> ()
          n153 = local write "Response"(w65) -> ()
          n154 = Build Array (concatenate)(w68, "iti mode") -> (w63:string[])
        }
      }
      n155 = Empty Array?(array=w34) -> (empty?=w33:bool)
    }
  }
  n156 = while {
    tunnel: w15 -> [w329]
    shift-right: [w325] -> w10
    shift-left: "State (in)" -> [w326]
    tunnel: w9 -> [w324]
    stop <- w328 stop-if-true
    # "MEASUREMENT THREAD"
    n157 = Wait on Notification(notifier=w329, ignore previous (F)=TRUE) -> (notification=w327:T24, error out=w328:errorcluster)  [unwired: 2 in, 2 out]
    n158 = Unbundle(w327) -> ("Params"=w323:T20, "Threshold Estimation"=w322:T19)
    n159 = case shown="No Error" w328 {
      tunnel: w323 -> [w342 _]
      tunnel: w326 -> [w352 w392]
      tunnel: [w348 w392] -> w325
      tunnel: w324 -> [w350 _]
      tunnel: w322 -> [w332 _]
      frame No Error {
        n160 = call "ABR-Initialize.vi"("Params"=w342, "State"=w352) -> ("Runtime"=w354:T29, "Analysis"=w351:T13, "Ceiling"=→"MAX SPL":dbl, "error out"=w355:errorcluster)  [unwired: 10 in]
        n161 = Unbundle By Name(w342) -> ("CAP or ABR"=w341:enum16{"CAP", "ABR"})
        n162 = while {
          shift-right: [w389] -> w340
          shift-left: w355 -> [w387]
          shift-right: [w385] -> _
          shift-left: w354 -> [w384]
          tunnel: w352 -> [w382]
          tunnel: [w381] -> w349
          shift-right: [w365] -> w338
          shift-left: w351 -> [w375]
          tunnel: w350 -> [w374]
          tunnel: ["NOTES"] -> w347
          tunnel: [w367] -> w346
          tunnel: [w366] -> w343
          tunnel: w342 -> [w366]
          tunnel: w341 -> [w364]
          tunnel: [w357] -> w331
          stop <- w391 stop-if-true
          # "stepsize"
          # "max SPL"
          # "array of levels"
          # "current SPL"
          n163 = call "ABR-Update Run Number.vi"("CAP or ABR"=w364, "State (in)"=w382) -> ("raw data filestem"=w357:path, "run #"=w358:i16, "State (out)"=w381:T16)  [unwired: 7 in]
          n164 = call "ABR-Set Level.vi"("Runtime"=w384, "error in (no error)"=w387) -> ("Runtime out"=w363:T29, "Level"=→"SPL":dbl, "error out"=w361:errorcluster)  [unwired: 11 in]
          n165 = call "ABR-Init Raw Data File.vi"("Runtime in"=w363, "Path"=w357, "error in (no error)"=w361) -> ("Runtime out"=w362:T29, "refnum out"=w359:refnum<file>, "error out"=w360:errorcluster)  [unwired: 10 in]
          n166 = control-ref of="Abort"() -> (w390:refnum<vi>)
          n167 = local write "Run #"(w358) -> ()
          n168 = call "ABR-Averager.vi"("Runtime"=w362, "Abort"=w390, "raw data file"=w359, "error in (no error)"=w360) -> ("Neural (uV)"=w380:dbl[], "microphonic (uV)"=w379:dbl[], "Averaging data"=w378:cluster{i32, i32}, "error out"=w383:errorcluster)  [unwired: 8 in]
          n169 = property on="Normalize traces" class="Bool (strict)"(error in=w383) -> (error out=w376:errorcluster, "Value"=w377:T18)  [unwired: 1 in, 1 out]
          n170 = call "ABR-Analyze.vi"("Neural (uV)"=w380, "Runtime"=w362, "microphonic (uV)"=w379, "Averaging data"=w378, "Normalize individual?"=w377, "error in"=w376, "Analysis"=w375, "Graphs"=w374) -> ("spread value"=w373:dbl, "Analysis out"=w365:T13, "error out"=w369:errorcluster)  [unwired: 5 in]
          n171 = property on="Abort" class="Bool (strict)"(error in=w369) -> (error out=w371:errorcluster, "Value"=w367:bool)  [unwired: 1 in, 1 out]
          n172 = property on="Analysis" class="Clust (strict)"("Val(Sgnl)"=w365) -> ()  [unwired: 2 in, 2 out]
          n173 = call "ABR-Adapt Number of Averages.vi"("Runtime"=w362, "Amplitude"=w373, "error in (no error)"=w371) -> ("Runtime out"=w372:T29, "error out"=w370:errorcluster)  [unwired: 11 in]
          n174 = call "ABR-Find Next Level.vi"("Runtime"=w372, "error in (no error)"=w370) -> ("Runtime out"=w385:T29, "Finished"=w388:bool, "error out"=w389:errorcluster)  [unwired: 11 in]
          n175 = Compound Arithmetic op=OR(w388, w367, w369) -> (w391:bool)
        }
        n176 = call "ABR-Estimate Threshold (wrapper).vi"("Threshold Estimation"=w332, "error in (no error)"=w340, "Analysis (in)"=w338) -> ("Analysis (out)"=w334:T13, "error out"=w339:errorcluster)  [unwired: 10 in, 1 out]
        n177 = Unbundle By Name(w334) -> ("threshold"=w336:dbl)
        n178 = call "ABR-Save Data.vi"("raw data filestem"=w331, "State (in)"=w349, "Params"=w343, "Aborted?"=w346, "error in (no error)"=w339, "Analysis"=w334, "Notes"=w347) -> ("State (out)"=w348:T16, "Datafile path"=w345:path, "Saved?"=w344:bool, "error out"=w335:errorcluster)  [unwired: 4 in, 1 out]
        n179 = property on="Analysis" class="Clust (strict)"(error in=w335, "Val(Sgnl)"=w334) -> (error out=w333:errorcluster)  [unwired: 1 in, 1 out]
        n180 = call "ABR3-Threshold To String.vi"("Threshold"=w336) -> ("String"=→"Thr":string)
        n181 = case shown="True" w344 {
          tunnel: w345 -> [_ w356]
          frame False {
          }
          frame True {
            "Datafile" <- w356
          }
        }
        n182 = property on="finished" class="Clust (strict)"("Val(Sgnl)"=w333) -> ()  [unwired: 2 in, 2 out]
      }
      frame Error {
      }
    }
  }
  "State" <- w10
